vi "TimeSimulator.vi"(8 "error in":errorcluster, 11 "Time Stamp":timestamp) -> (0 "error in 2":errorcluster, 2 "AppliedBoosterDosage":T1, 3 "BoosterDoseTriggerred":bool)   [LabVIEW 2019]
uses:
  DrugDosageTimeStampReference.ctl
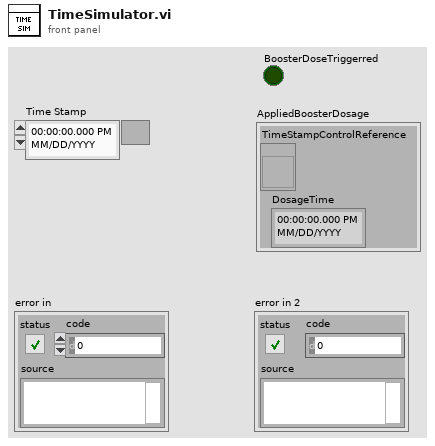
[diagram p1: front panel]
types:
  T1 = typedef "DrugDosageTimeStampReference.ctl" = cluster{"TimeStampControlReference":refnum<vi>, "DosageTime":timestamp}
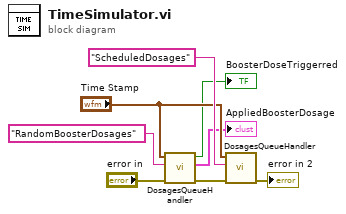
[diagram p0: block diagram]
diagram:
  n1 = call "DosagesQueueHandler.vi"("error in (no error)"="error in", "DosagesQueueName"="RandomBoosterDosages" ("name (unnamed)"), "CurrentTime"="Time Stamp") -> ("error out"=w2:errorcluster, "AppliedDosage"=→"AppliedBoosterDosage":T1, "Sucess"=→"BoosterDoseTriggerred":bool)  [unwired: 6 in]
  n2 = call "DosagesQueueHandler.vi"("error in (no error)"=w2, "DosagesQueueName"="ScheduledDosages" ("name (unnamed)"), "CurrentTime"="Time Stamp") -> ("error out"=→"error in 2":errorcluster)  [unwired: 6 in, 2 out]
